vi "parse_camera_dimensions.vi"(1 "String":string="2048, 0") -> (0 "Camera Dimensions Out":dbl[](array[numeric]))   [LabVIEW 2017]
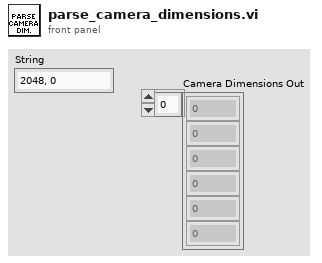
[diagram p1: front panel]
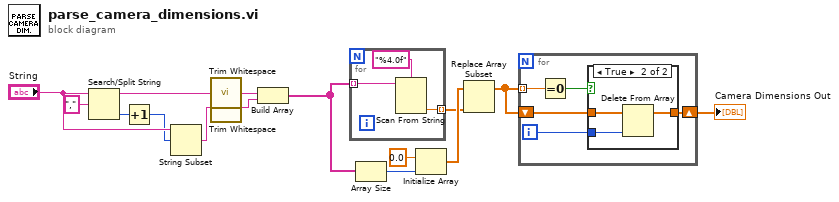
[diagram p0: block diagram]
diagram:
  n1 = Search/Split String(string="String", search string/char (-)=",") -> (substring before match=w14:string, offset of match=w12:i32)  [unwired: 1 in, 1 out]
  n2 = Increment(x=w12) -> (x+1=w11:i32)
  n3 = String Subset(string="String", offset (0)=w11) -> (substring=w10:string)  [unwired: 1 in]
  n4 = call <vilib>:"Trim Whitespace.vi"("string"=w14) -> ("trimmed string"=w9:string)  [unwired: 1 in]
  n5 = call <vilib>:"Trim Whitespace.vi"("string"=w10) -> ("trimmed string"=w8:string)  [unwired: 1 in]
  n6 = Build Array(w9, w8) -> (w7:string[])
  n7 = for {
    tunnel: w7 -> [w17] mode=indexing
    tunnel: [w18] -> w3 mode=indexing
    n8 = Scan From String(format string="%4.0f", input string=w17) -> (output 1=w18:dbl)  [unwired: 3 in, 3 out]
  }
  n9 = Array Size(array=w7) -> (size(s)=w6:i32)
  n10 = Initialize Array(0.0 ("element"), w6) -> (w5:dbl[])
  n11 = Replace Array Subset(array=w5, new element=w3) -> (w2:dbl[])  [unwired: 1 in]
  n12 = for {
    tunnel: w2 -> [w23] mode=indexing
    shift-right: [w19] -> w1
    shift-left: w2 -> [w21]
    i -> [w20]
    n13 = Equal To 0?(x=w23) -> (x = 0?=w22:bool)
    n14 = case shown="True" w22 {
      tunnel: w21 -> [w24 w27]
      tunnel: w20 -> [_ w26]
      tunnel: [w24 w25] -> w19
      frame False {
      }
      frame True {
        n15 = Delete From Array(array=w27, index=w26) -> (array with subset deleted=w25:dbl[])  [unwired: 1 in, 1 out]
      }
    }
  }
  "Camera Dimensions Out" <- w1
